vi "Read QuotesOnTableName.vi"(8 "error in (no error)":errorcluster, 11 "SqliteConnection in":refnum<class "DBC.lvclass">) -> (0 "error out":errorcluster, 2 "QuotesOnTableName":bool, 3 "SqliteConnection out":refnum<class "DBC.lvclass">)   [LabVIEW 2020, in "ORM_DBC_Sqlite.lvlib" / "DBC.lvclass"]
uses:
  DBC.lvclass
  DBC.lvclass/DBC.ctl
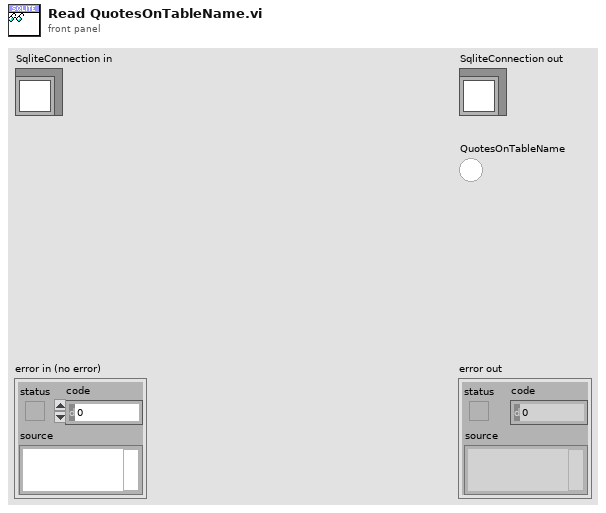
[diagram p1: front panel]
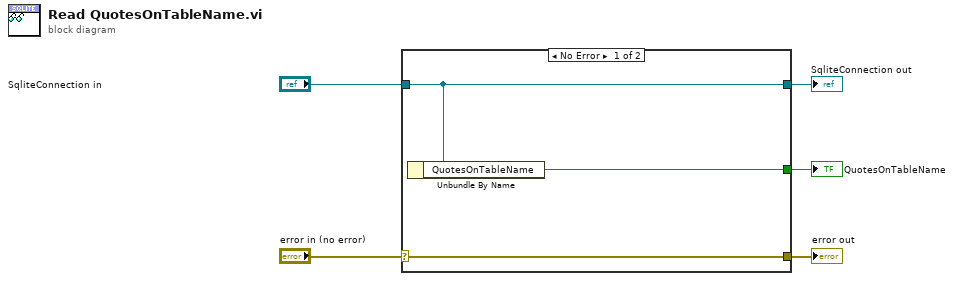
[diagram p0: block diagram]
diagram:
  n1 = case shown="No Error" "error in (no error)" {
    selector: "error in (no error)" -> [w8 w9]
    tunnel: [w8 w9] -> w4
    tunnel: [w7 w10] -> w2
    tunnel: "SqliteConnection in" -> [w7 w10]
    tunnel: [w6 _] -> w1
    frame No Error {
      n2 = Unbundle By Name(w7) -> ("QuotesOnTableName"=w6:bool)
    }
    frame Error {
    }
  }
  "error out" <- w4
  "SqliteConnection out" <- w2
  "QuotesOnTableName" <- w1
